vi "Make Directory Tree.vi"(8 "error in (no error)":errorcluster, 11 "Path":path=path "") -> (0 "error out":errorcluster, 3 "Created Directory":path)   [LabVIEW 2017, in "CL_G3_VIComponentBuilder.lvlib"]
uses:
  CL_G3_VIComponentBuilder.lvlib
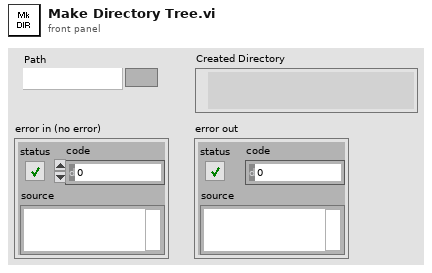
[diagram p1: front panel]
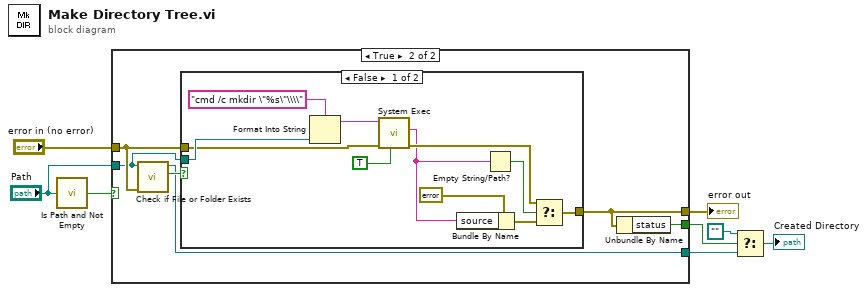
[diagram p0: block diagram]
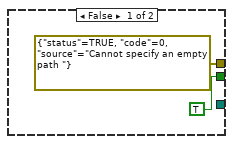
[diagram p2: hidden frame]
diagram:
  n1 = call <vilib>:"Is Path and Not Empty.vi"("path"="Path") -> ("Is Path and Not Empty?"=w2:bool)  [unwired: 4 in]
  n2 = case shown="True" w2 {
    tunnel: "error in (no error)" -> [_ w15]
    tunnel: [TRUE ("status") w14] -> w7
    tunnel: [_ w13] -> w6
    tunnel: "Path" -> [_ w12]
    tunnel: [errorcluster {"status"=TRUE, "code"=0, "source"="Cannot specify an empty path "} ("error in (no error)") w11] -> w1
    frame False {
    }
    frame True {
      n3 = call <vilib>:"Check if File or Folder Exists.vi"("error in (no error)"=w15, "path"=w12) -> ("file or folder exists?"=w16:bool, "dup path"=w13:path)  [unwired: 7 in, 1 out]
      n4 = case shown="False" w16 {
        tunnel: w12 -> [w27 _]
        tunnel: [w17 w28] -> w11
        tunnel: w15 -> [w26 w28]
        frame False {
          n5 = Format Into String(format string="cmd /c mkdir \"%s\"\\\\", w27) -> (resulting string=w24:string)  [unwired: 2 in, 1 out]
          n6 = call <vilib>:"System Exec.vi"("run minimized? (F)"=TRUE, "error in (no error)"=w26, "command line"=w24) -> ("error out"=w22:errorcluster, "standard error"=w18:string)  [unwired: 5 in, 2 out]
          n7 = Bundle By Name(cluster=errorcluster {"status"=TRUE, "code"=0, "source"=""} ("error out"), "source"=w18) -> (w20:errorcluster)
          n8 = Empty String/Path?(string/path=w18) -> (empty?=w21:bool)
          n9 = Select(t=w22, s=w21, f=w20) -> (s? t:f=w17:errorcluster)
        }
        frame True {
        }
      }
      n10 = Unbundle By Name(w11) -> ("status"=w14:bool)
    }
  }
  "error out" <- w1
  n11 = Select(t=path "", s=w7, f=w6) -> (s? t:f=→"Created Directory":path)
